vi "movearea.vi"(8 "error in (no error)":errorcluster, 11 "Input":string="y-") -> (0 "error out":errorcluster, 3 "Output":string)   [LabVIEW 2014]
uses:
  <userlib>/Nanonis Prog Interface V5/Nanonis Prog Interface.lvlib
panel:
  in  "STMStatus":T1 {"Size (m)"."Height" format="%.2p"; "Size (m)"."Width" format="%.2p"; "Current (A)" format="%#_6p"; "Z position (m)" format="%#_6p"; "Center coordinates (m)"."Yc" format="%.2p"; "Center coordinates (m)"."Xc" format="%.2p"}
  out "size(s)":i32=3
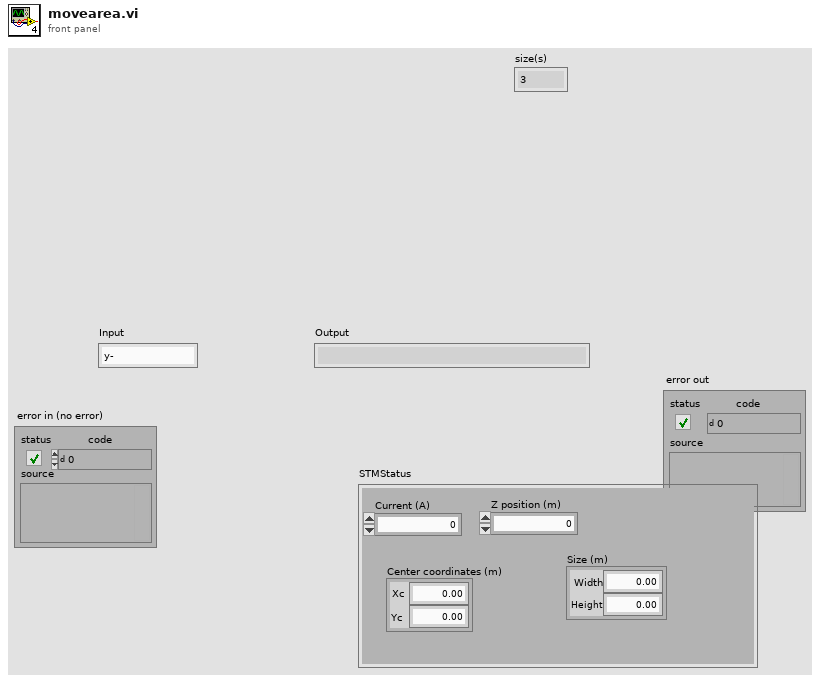
[diagram p1: front panel]
types:
  T1 = cluster{"Center coordinates (m)":cluster{"Xc":sgl, "Yc":sgl}, "Z position (m)":sgl, "Current (A)":sgl, "Size (m)":cluster{"Width":sgl, "Height":sgl}}
  T2 = enum8{"Group 1", "Group 2", "Group 3", "Group 4", "Group 5", "Group 6"}
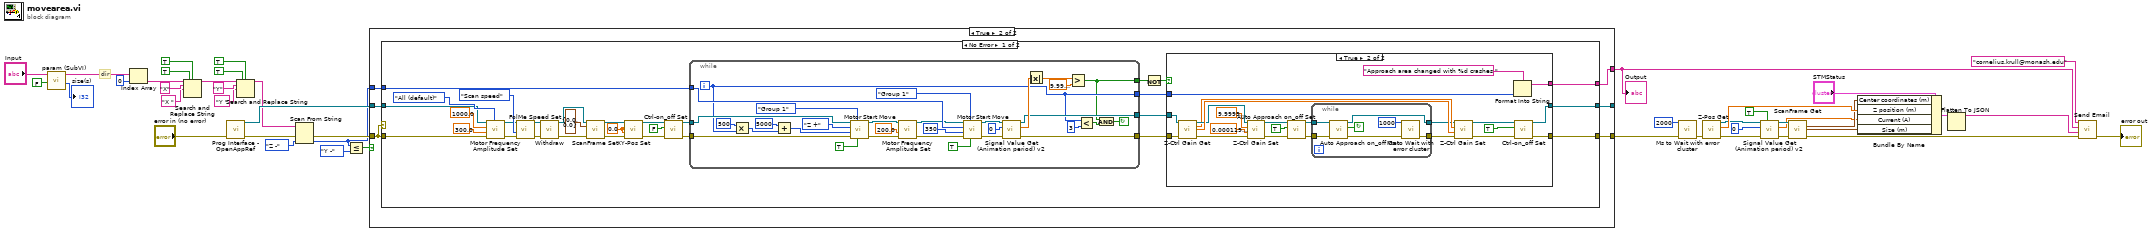
[diagram p0: block diagram]
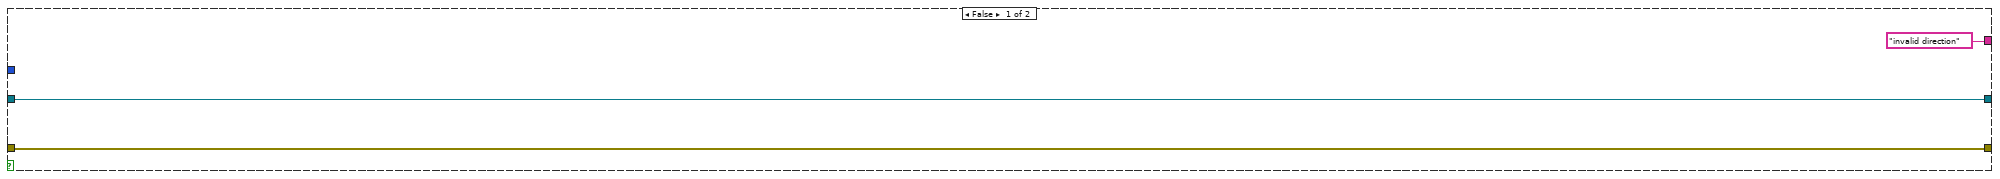
[diagram p2: hidden frame]
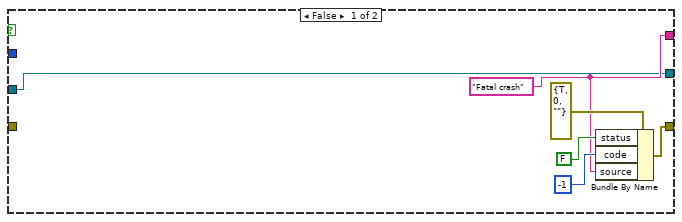
[diagram p3: hidden frame]
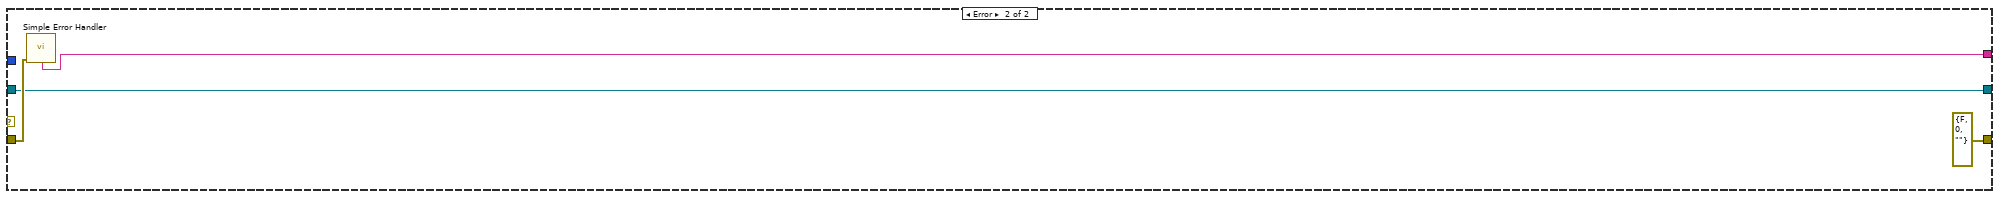
[diagram p4: hidden frame]
diagram:
  # "dir"
  n1 = call <userlib>:"param (SubVI).vi"("Numeric"=FALSE, "Input"="Input") -> ("num"=→"size(s)":i32, "Array"=w40:string[])  [unwired: 7 in, 1 out]
  n2 = Index Array(array=w40, index=0) -> (element=w31:string)
  n3 = Search and Replace String(replace all?=TRUE ("replace all? (F)"), case sensitive?=TRUE ("ignore case? (F)"), input string=w31, search string="X", replace string="X " ("replace string (\"\")")) -> (result string=w22:string)  [unwired: 3 in, 3 out]
  n4 = call <userlib>:"Prog Interface - OpenAppRef.vi"("Error in (no error)"="error in (no error)") -> ("Error out"=w37:errorcluster, "Application reference"=w41:refnum<vi>)  [unwired: 5 in]
  n5 = Search and Replace String(replace all?=TRUE ("replace all? (F)"), case sensitive?=TRUE ("ignore case? (F)"), input string=w22, search string="Y", replace string="Y " ("replace string (\"\")")) -> (result string=w21:string)  [unwired: 3 in, 3 out]
  n6 = Scan From String(input string=w21, error in=w37, default 1=enum16{"X +", "X -", "Y +", "Y -", "Z +", "Z -"}."Z -" ("Direction")) -> (error out=w36:errorcluster, output 1=w35:enum16{"X +", "X -", "Y +", "Y -", "Z +", "Z -"})  [unwired: 2 in, 2 out]
  n7 = Less Or Equal?(x=w35, y=enum16{"X +", "X -", "Y +", "Y -", "Z +", "Z -"}."Y -") -> (x <= y?=w33:bool)
  n8 = case shown="True" w33 {
    tunnel: w41 -> [w45 w53]
    tunnel: w35 -> [_ w52]
    tunnel: w36 -> [w47 w51]
    tunnel: [w47 w50] -> w5
    tunnel: ["invalid direction" ("message") w49] -> w16
    tunnel: [w45 w48] -> _
    frame False {
    }
    frame True {
      n9 = case shown="No Error" w51 {
        tunnel: w53 -> [w71 w151]
        tunnel: w52 -> [w69 _]
        tunnel: w51 -> [w68 w154]
        tunnel: [w55 errorcluster {"status"=FALSE, "code"=0, "source"=""} ("error out")] -> w50
        tunnel: [w60 w153] -> w49
        tunnel: [w54 w151] -> w48
        frame No Error {
          w78 = sgl 0.0 ("X (m)")
          n10 = call <userlib>:"Motor Frequency Amplitude Set.vi"("Axis (All)"=enum16{"All (default)", "X", "Y", "Z"}."All (default)", "Error in (no error)"=w68, "Amplitude (V) (NaN=no change)"=sgl 300.0, "Frequency (Hz) (NaN=no change)"=sgl 1000.0, "Application ref in"=w71) -> ("Error out"=w67:errorcluster, "Application ref out"=w70:refnum<vi>)  [unwired: 5 in]
          n11 = call <userlib>:"FolMe Speed Set.vi"("error in (no error)"=w67, "Speed Setting (Custom)"=enum32{"Scan speed", "Custom speed"}."Scan speed", "Application ref in"=w70) -> ("error out"=w75:errorcluster, "Application ref out"=w76:refnum<vi>)  [unwired: 5 in]
          n12 = call <userlib>:"Withdraw.vi"("Error in (no error)"=w75, "Application ref in"=w76) -> ("Error out"=w82:errorcluster, "Application ref out"=w83:refnum<vi>)  [unwired: 8 in]
          n13 = call <userlib>:"ScanFrame Set.vi"("Application ref in"=w83, "Center coordinates (m)"=cluster{"Xc":sgl, "Yc":sgl} {"Xc"=0.0, "Yc"=0.0}, "error in (no error)"=w82) -> ("Application ref out"=w79:refnum<vi>, "error out"=w80:errorcluster)  [unwired: 11 in]
          n14 = call <userlib>:"XY-Pos Set.vi"("error in (no error)"=w80, "Y (m)"=w78, "X (m)"=w78, "Application ref in"=w79) -> ("error out"=w61:errorcluster, "Application ref out"=w62:refnum<vi>)  [unwired: 4 in]
          n15 = call <userlib>:"Ctrl-on_off Set.vi"("error in (no error)"=w61, "Z Controller ON/OFF"=FALSE, "Application ref in"=w62) -> ("error out"=w63:errorcluster, "Application ref out"=w64:refnum<vi>)  [unwired: 7 in]
          n16 = while {
            tunnel: w69 -> [w150]
            tunnel: [w130] -> w66
            tunnel: [w129] -> w65
            tunnel: w64 -> [w128]
            tunnel: w63 -> [w127]
            tunnel: [w126] -> w59
            tunnel: [w125] -> w58
            i -> [w126]
            stop <- w132 continue-if-true
            n17 = Multiply(x=500, y=w126) -> (x*y=w135:i32)
            n18 = Add(x=u16 5000 ("Number of steps"), y=w135) -> (x+y=w137:i32)
            n19 = call <userlib>:"Motor Start Move.vi"("Wait until finished? (F)"=TRUE, "Group"=T2."Group 1", "Error in (no error)"=w127, "Number of steps"=w137, "Direction"=enum16{"X +", "X -", "Y +", "Y -", "Z +", "Z -"}."Z +", "Application ref in"=w128) -> ("Error out"=w121:errorcluster, "Application ref out"=w124:refnum<vi>)  [unwired: 3 in]
            n20 = call <userlib>:"Motor Frequency Amplitude Set.vi"("Error in (no error)"=w121, "Amplitude (V) (NaN=no change)"=sgl 200.0, "Application ref in"=w124) -> ("Error out"=w122:errorcluster, "Application ref out"=w123:refnum<vi>)  [unwired: 7 in]
            n21 = call <userlib>:"Motor Start Move.vi"("Wait until finished? (F)"=TRUE, "Group"=T2."Group 1", "Error in (no error)"=w122, "Number of steps"=u16 350, "Direction"=w150, "Application ref in"=w123) -> ("Error out"=w141:errorcluster, "Application ref out"=w143:refnum<vi>)  [unwired: 3 in]
            n22 = call <userlib>:"Signal Value Get (Animation period) v2.vi"("error in (no error)"=w141, "Signal index (0-79)"=i8 0, "Application ref in"=w143) -> ("error out"=w129:errorcluster, "Signal value"=w140:sgl, "Application ref out"=w130:refnum<vi>)  [unwired: 5 in]
            n23 = Absolute Value(x=w140) -> (abs(x)=w138:sgl)
            n24 = Greater?(x=w138, y=sgl 1e-09) -> (0:w125:bool)
            n25 = Less?(x=w126, y=3) -> (x < y?=w131:bool)
            n26 = And(x=w125, y=w131) -> (x .and. y?=w132:bool)
          }
          n27 = Not(x=w58) -> (.not. x?=w57:bool)
          n28 = case shown="True" w57 {
            tunnel: w66 -> [w84 w112]
            tunnel: w65 -> [_ w102]
            tunnel: [w86 w94] -> w60
            tunnel: w59 -> [_ w93]
            tunnel: [w85 w91] -> w55
            tunnel: [w84 w90] -> w54
            frame False {
              w86 = "Fatal crash"
              n29 = Bundle By Name(cluster=errorcluster {"status"=TRUE, "code"=0, "source"=""} ("error out"), "status"=FALSE, "code"=-1, "source"=w86) -> (w85:errorcluster)
            }
            frame True {
              n30 = call <userlib>:"Z-Ctrl Gain Get.vi"("Application ref in"=w112, "error in (no error)"=w102) -> ("Application ref out"=w108:refnum<vi>, "P-gain"=w106:sgl, "Time constant (s)"=w111:sgl, "error out"=w101:errorcluster)  [unwired: 9 in, 1 out]
              n31 = call <userlib>:"Z-Ctrl Gain Set.vi"("error in (no error)"=w101, "Time constant (s)"=sgl 0.00012, "P-gain"=sgl 1e-11, "Application ref in"=w108) -> ("error out"=w100:errorcluster, "Application ref out"=w107:refnum<vi>)  [unwired: 5 in]
              n32 = call <userlib>:"Auto Approach on_off Set.vi"("Error in (no error)"=w100, "Auto approach start/stop (F)"=TRUE, "Application ref in"=w107) -> ("Error out"=w99:errorcluster, "Application ref out"=w104:refnum<vi>)  [unwired: 5 in]
              n33 = while {
                tunnel: w104 -> [w116]
                tunnel: [w115] -> w103
                tunnel: w99 -> [w114]
                tunnel: [w113] -> w98
                stop <- w119 continue-if-true
                n34 = call <userlib>:"Auto Approach on_off Get.vi"("Error in (no error)"=w114, "Application ref in"=w116) -> ("Error out"=w117:errorcluster, "Auto approach on/off status"=w119:bool, "Application ref out"=w115:refnum<vi>)  [unwired: 5 in]
                n35 = call <userlib>:"Ms to Wait with error cluster.vi"("error in (no error)"=w117, "milliseconds to wait"=u32 1000) -> ("error out"=w113:errorcluster)  [unwired: 4 in, 1 out]
              }
              n36 = call <userlib>:"Z-Ctrl Gain Set.vi"("error in (no error)"=w98, "Time constant (s)"=w111, "P-gain"=w106, "Application ref in"=w103) -> ("error out"=w95:errorcluster, "Application ref out"=w97:refnum<vi>)  [unwired: 5 in]
              n37 = Format Into String(format string="Approach area changed with %d crashes " ("initial string"), w93) -> (resulting string=w94:string)  [unwired: 2 in, 1 out]
              n38 = call <userlib>:"Ctrl-on_off Set.vi"("error in (no error)"=w95, "Z Controller ON/OFF"=TRUE, "Application ref in"=w97) -> ("error out"=w91:errorcluster, "Application ref out"=w90:refnum<vi>)  [unwired: 7 in]
            }
          }
        }
        frame Error {
          n39 = call <vilib>:"Simple Error Handler.vi"("error in (no error)"=w154) -> ("message"=w153:string)  [unwired: 4 in, 4 out]
        }
      }
    }
  }
  "Output" <- w16
  n40 = call <userlib>:"Ms to Wait with error cluster.vi"("error in (no error)"=w5, "milliseconds to wait"=u32 2000) -> ("error out"=w4:errorcluster)  [unwired: 4 in, 1 out]
  n41 = call <userlib>:"Z-Pos Get.vi"("error in (no error)"=w4) -> ("error out"=w9:errorcluster, "Z position (m)"=w15:sgl, "Application ref out"=w12:refnum<vi>)  [unwired: 8 in]
  n42 = call <userlib>:"Signal Value Get (Animation period) v2.vi"("Wait for newest data (F=False)"=TRUE, "error in (no error)"=w9, "Signal index (0-79)"=i8 0, "Application ref in"=w12) -> ("error out"=w10:errorcluster, "Signal value"=w7:sgl, "Application ref out"=w11:refnum<vi>)  [unwired: 4 in]
  n43 = call <userlib>:"ScanFrame Get.vi"("Application ref in"=w11, "error in (no error)"=w10) -> ("Center coordinates (m)"=w14:cluster{"Xc":sgl, "Yc":sgl}, "Size (m)"=w13:cluster{"Width":sgl, "Height":sgl}, "error out"=w2:errorcluster)  [unwired: 9 in, 2 out]
  n44 = Bundle By Name(cluster="STMStatus", "Center coordinates (m)"=w14, "Z position (m)"=w15, "Current (A)"=w7, "Size (m)"=w13) -> (w18:T1)
  n45 = Flatten To JSON(anything=w18) -> (JSON string=w17:string)  [unwired: 2 in, 1 out]
  n46 = call "Send Email"("error in"=w2, "Message"=w17, "Subject"=w16, "Recipients"="cornelius.krull@monash.edu") -> ("error out"=→"error out":errorcluster)  [unwired: 7 in]
